vi "Set volume table.vi"(8 "error in (no error)":errorcluster, 10 "Volume map in":dbl[][](array[numeric]), 11 "Tomo in":refnum<class "Tomo.lvclass">) -> (0 "error out":errorcluster, 3 "Tomo out":refnum<class "Tomo.lvclass">)   [LabVIEW 2012, in "Tomo.lvclass"]
uses:
  Tomo.lvclass
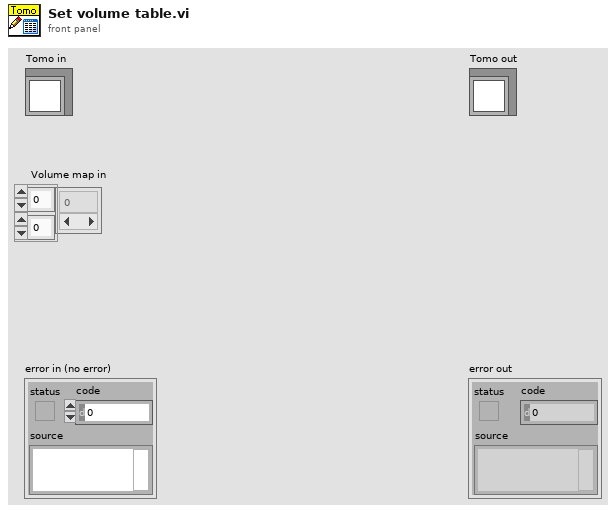
[diagram p1: front panel]
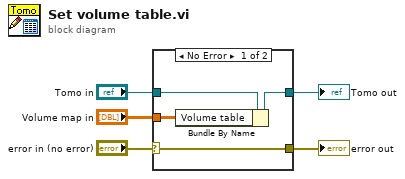
[diagram p0: block diagram]
diagram:
  n1 = case shown="No Error" "error in (no error)" {
    selector: "error in (no error)" -> [w9 w11]
    tunnel: [w9 w11] -> w4
    tunnel: [w6 w10] -> w2
    tunnel: "Tomo in" -> [w7 w10]
    tunnel: "Volume map in" -> [w8 _]
    frame No Error {
      n2 = Bundle By Name(cluster=w7, "Volume table"=w8) -> (w6:refnum<class "Tomo.lvclass">)
    }
    frame Error {
    }
  }
  "error out" <- w4
  "Tomo out" <- w2
